vi "Auto Calibrate.vi"() -> ()   [LabVIEW 2013]
uses:
  Reload Pro/Reload-pro.lvclass
panel:
  in  "Current (mA)":dbl
  in  "VISA resource name":refnum<visa-resource-name>
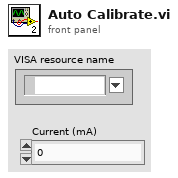
[diagram p1: front panel]
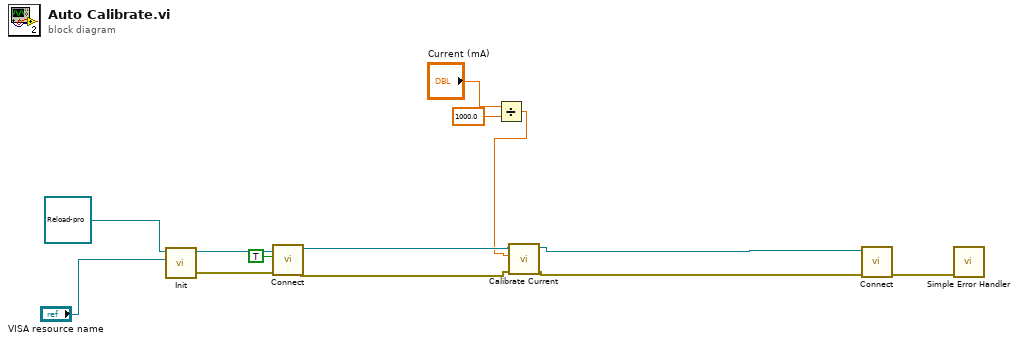
[diagram p0: block diagram]
diagram:
  n1 = call-dynamic "Init.vi"("VISA resource name"="VISA resource name", "Reload-pro in"=refnum<class "Reload-pro.lvclass"> refnum ("Reload-pro.lvclass")) -> ("error out"=w10:errorcluster, "Reload-pro out"=w11:refnum<class "Reload-pro.lvclass">)  [unwired: 8 in]
  n2 = call-dynamic "Connect.vi"("error in (no error)"=w10, "Connect?"=TRUE, "Reload-pro in"=w11) -> ("error out"=w5:errorcluster, "Reload-pro out"=w6:refnum<class "Reload-pro.lvclass">)  [unwired: 7 in]
  n3 = Divide(x="Current (mA)", y=1000.0) -> (x/y=w1:dbl)
  n4 = call-dynamic "Calibrate Current.vi"("error in (no error)"=w5, "Current (A)"=w1, "Reload-pro in"=w6) -> ("error out"=w4:errorcluster, "Reload-pro out"=w7:refnum<class "Reload-pro.lvclass">)  [unwired: 7 in]
  n5 = call-dynamic "Connect.vi"("error in (no error)"=w4, "Reload-pro in"=w7) -> ("error out"=w8:errorcluster)  [unwired: 8 in, 1 out]
  n6 = call <vilib>:"Simple Error Handler.vi"("error in (no error)"=w8) -> ()  [unwired: 4 in, 5 out]
